vi "Execute Industrial Controllers.vi"(8 "error in (no error)":errorcluster, 11 "State Variables in":T1 {"Config"."Config"."Industrial Settings"."Write Refs"."Data Reference" format="%.0x"; "Config"."Config"."Industrial Settings"."Read Refs"."Data Reference" format="%.0x"; "Config"."Config"."PID Settings"."Read Refs"."Data Reference" format="%.0x"; "Config"."Config"."PID Settings"."Write Refs"."Data Reference" format="%.0x"}) -> (0 "error out":errorcluster, 3 "State Variables out":T1 {"Config"."Config"."Industrial Settings"."Write Refs"."Data Reference" format="%.0x"; "Config"."Config"."Industrial Settings"."Read Refs"."Data Reference" format="%.0x"; "Config"."Config"."PID Settings"."Read Refs"."Data Reference" format="%.0x"; "Config"."Config"."PID Settings"."Write Refs"."Data Reference" format="%.0x"})   [LabVIEW 2015, in "Control Addon Engine.lvlib"]
uses:
  Control Addon Engine.lvlib
  Types/RT Driver State Variables.ctl
  <vilib>/NI/NIVS Inline Async API/_VS Inline Async API/VS Inline Async API/VS Inline Async API.lvclass
  Types/RT Configuration.ctl
  Shared/Types/Gain Schedule.ctl
  Shared/Types/Compiled Settings.ctl
  Shared/Types/Compiled PID Settings.ctl
  <vilib>/NI Veristand/Custom Device API/Block Data Reference.ctl
  <vilib>/NI Veristand/Custom Device API/Data Reference.ctl
  Shared/Types/Compiled Industrial Settings.ctl
  Shared/Types/Compiled Industrial Parameters.ctl
  <vilib>/NI Veristand/Custom Device API/Global Data Refs.vi
  <vilib>/NI VeriStand/Custom Device API/Custom Device API.lvlib
  Shared/Control Addon Shared.lvlib
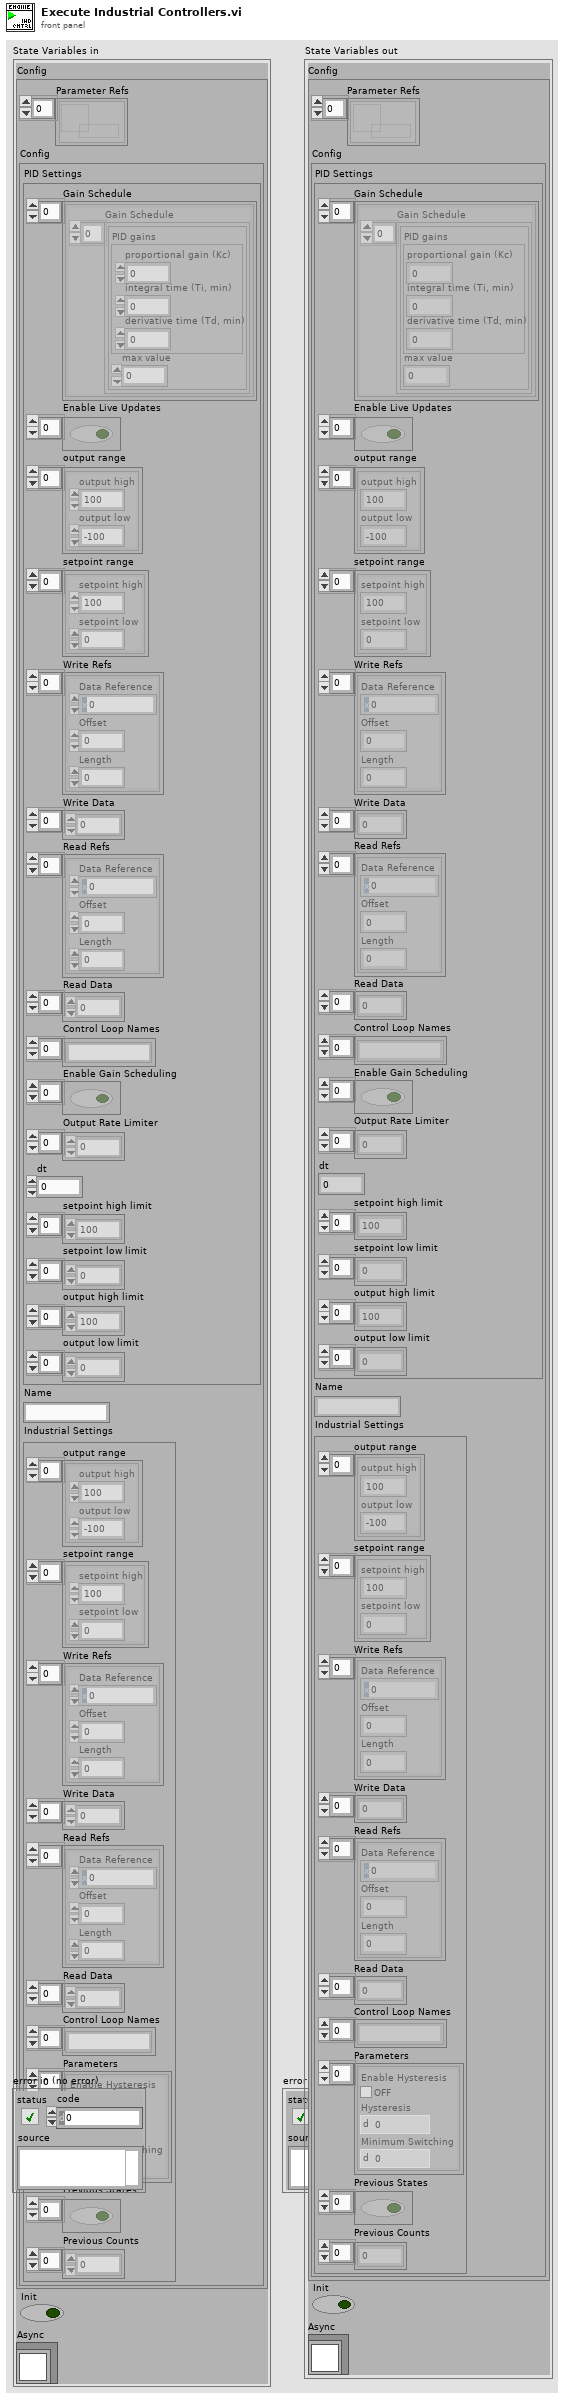
[diagram p1: front panel]
types:
  T1 = typedef "Control Addon Engine.lvlib/RT Driver State Variables.ctl" = cluster{"Config":T2, "Init":bool, "Async":refnum<class "VS Inline Async API.lvclass">}
  T2 = typedef "Control Addon Engine.lvlib/RT Configuration.ctl" = cluster{"Parameter Refs":refnum<data-value>[], "Config":T3}
  T3 = typedef "Control Addon Shared.lvlib/Compiled Settings.ctl" = cluster{"PID Settings":T4, "Name":string, "Industrial Settings":T8}
  T4 = typedef "Control Addon Shared.lvlib/Compiled PID Settings.ctl" = cluster{"Gain Schedule":T5[], "Enable Live Updates":bool[], "output range":cluster{"output high":dbl, "output low":dbl}[], "setpoint range":cluster{"setpoint high":dbl, "setpoint low":dbl}[], "Write Refs":T6[], "Write Data":dbl[], "Read Refs":T6[], "Read Data":dbl[], "Control Loop Names":string[], "Enable Gain Scheduling":bool[], "Output Rate Limiter":dbl[], "dt":dbl, "setpoint high limit":dbl[], "setpoint low limit":dbl[], "output high limit":dbl[], "output low limit":dbl[]}
  T5 = typedef "Control Addon Shared.lvlib/Gain Schedule.ctl" = cluster{"Gain Schedule":cluster{"PID gains":cluster{"proportional gain (Kc)":dbl, "integral time (Ti, min)":dbl, "derivative time (Td, min)":dbl}, "max value":dbl}[]}
  T6 = typedef "Custom Device API.lvlib/Block Data Reference.ctl" = cluster{"Data Reference":T7, "Offset":u64, "Length":u64}
  T7 = typedef "Custom Device API.lvlib/Data Reference.ctl" = i32
  T8 = typedef "Control Addon Shared.lvlib/Compiled Industrial Settings.ctl" = cluster{"output range":cluster{"output high":dbl, "output low":dbl}[], "setpoint range":cluster{"setpoint high":dbl, "setpoint low":dbl}[], "Write Refs":T6[], "Write Data":dbl[], "Read Refs":T6[], "Read Data":dbl[], "Control Loop Names":string[], "Parameters":T9[], "Previous States":bool[], "Previous Counts":u64[]}
  T9 = typedef "Control Addon Shared.lvlib/Compiled Industrial Parameters.ctl" = cluster{"Enable Hysteresis":bool, "Hysteresis":dbl, "Minimum Switching":u64}
  T10 = cluster{"setpoint high":dbl, "setpoint low":dbl}[]
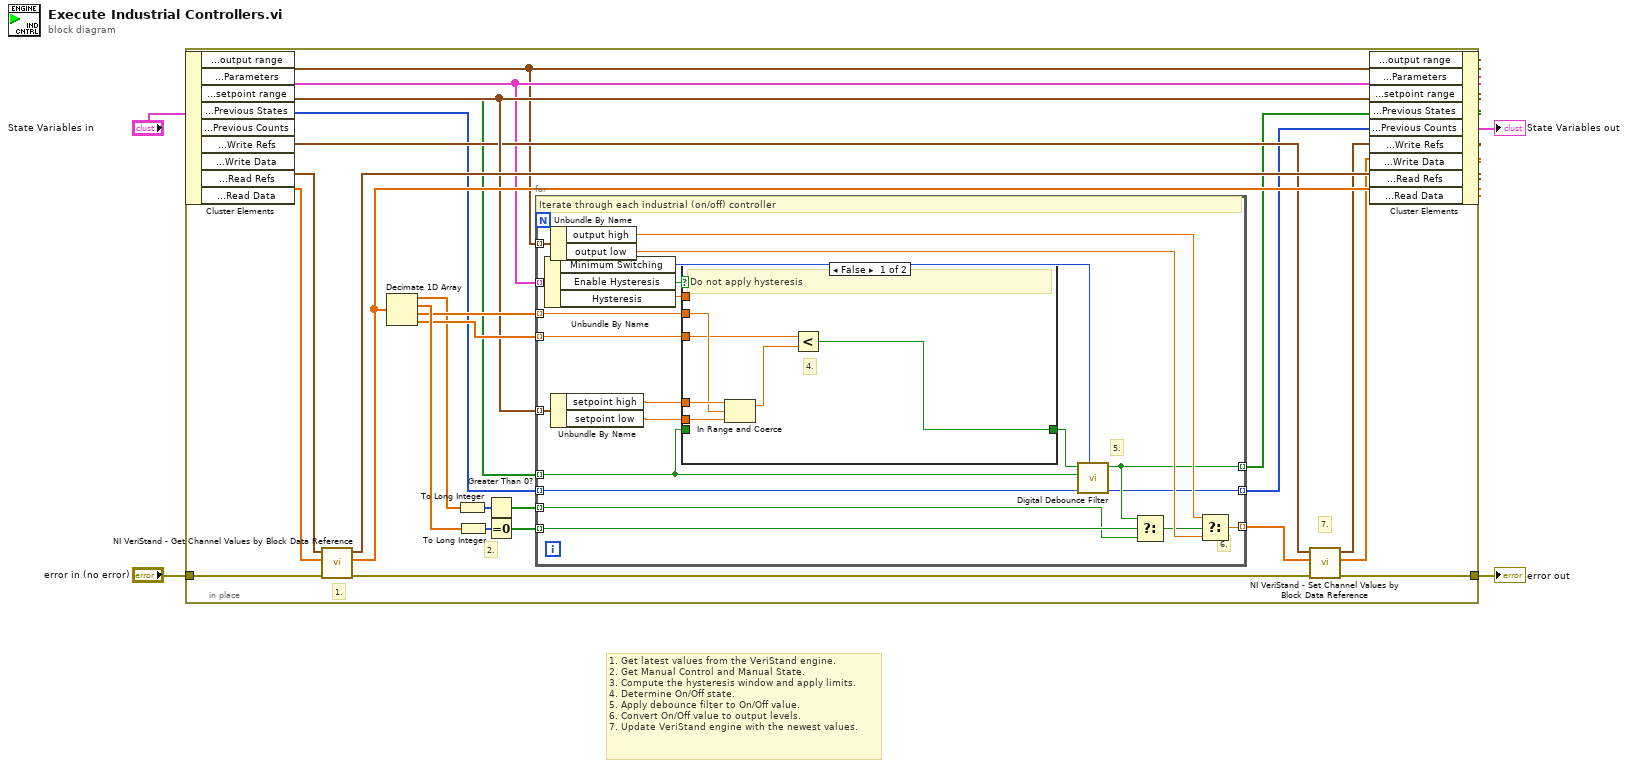
[diagram p0: block diagram]
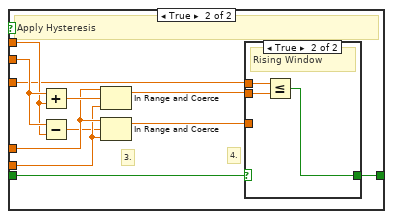
[diagram p2: hidden frame]
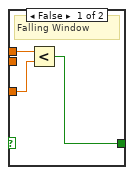
[diagram p3: hidden frame]
diagram:
  # "1. Get latest values from the VeriStand engine.\n2. Get Manual Control and Manual State.\n3. Compute the hysteresis window and apply limits.\n4. Determine On/Off state.\n5. Apply debounce filter to On/Off value.\n6. Convert On/Off value to output levels.\n7. Update VeriStand engine with the newest values."
  n1 = in-place {
    in-place-border: "error in (no error)" -> [w30]
    in-place-border: [w18] -> w4
    # "7."
    # "2."
    # "1."
    n2 = in-place-cluster #1("State Variables in") -> ("Config.Config.Industrial Settings.output range"=w5:cluster{"output high":dbl, "output low":dbl}[], "Config.Config.Industrial Settings.Parameters"=w10:T9[], "Config.Config.Industrial Settings.setpoint range"=w19:T10, "Config.Config.Industrial Settings.Previous States"=w9:bool[], "Config.Config.Industrial Settings.Previous Counts"=w8:u64[], "Config.Config.Industrial Settings.Write Refs"=w17:T6[], "Config.Config.Industrial Settings.Read Refs"=w29:T6[], "Config.Config.Industrial Settings.Read Data"=w28:dbl[])  [unwired: 1 out]
    n3 = call <vilib>:"NI VeriStand - Get Channel Values by Block Data Reference.vi"("error in (no error)"=w30, "Values Array in"=w28, "Block Data Ref"=w29) -> ("error out"=w25:errorcluster, "Values Array out"=w24:dbl[], "Block Data Ref dup"=w26:T6[])  [unwired: 6 in]
    n4 = Decimate 1D Array(w24) -> (w12:dbl[], w22:dbl[], w21:dbl[], w20:dbl[])
    n5 = To Long Integer(number=w12) -> (32bit integer=w13:i32[])
    n6 = To Long Integer(number=w22) -> (32bit integer=w27:i32[])
    n7 = Greater Than 0?(x=w13) -> (x > 0?=w11:bool[])
    n8 = Equal To 0?(x=w27) -> (x = 0?=w23:bool[])
    n9 = for {
      tunnel: w11 -> [w48] mode=indexing
      tunnel: w23 -> [w51] mode=indexing
      tunnel: w21 -> [w42] mode=indexing
      tunnel: w20 -> [w38] mode=indexing
      tunnel: w19 -> [w50] mode=indexing
      tunnel: w5 -> [w49] mode=indexing
      tunnel: [w44] -> w14 mode=indexing
      tunnel: w10 -> [w43] mode=indexing
      tunnel: w9 -> [w34] mode=indexing
      tunnel: [w36] -> w7 mode=indexing
      tunnel: w8 -> [w33] mode=indexing
      tunnel: [w32] -> w6 mode=indexing
      # "6."
      # "5."
      # "Iterate through each industrial (on/off) controller"
      n10 = Unbundle By Name(w43) -> ("Minimum Switching"=w31:u64, "Enable Hysteresis"=w37:bool, "Hysteresis"=w41:dbl)
      n11 = Unbundle By Name(w49) -> ("output high"=w46:dbl, "output low"=w47:dbl)
      n12 = Unbundle By Name(w50) -> ("setpoint high"=w40:dbl, "setpoint low"=w39:dbl)
      n13 = case shown="False" w37 {
        tunnel: w42 -> [w55 w68]
        tunnel: w41 -> [_ w67]
        tunnel: w40 -> [w57 w65]
        tunnel: w39 -> [w56 w64]
        tunnel: w38 -> [w53 w62]
        tunnel: [w52 w61] -> w35
        tunnel: w34 -> [_ w58]
        frame False {
          # "4."
          # "Do not apply hysteresis"
          n14 = In Range and Coerce(upper limit=w57, x=w55, lower limit=w56) -> (coerced(x)=w54:dbl)  [unwired: 1 out]
          n15 = Less?(x=w53, y=w54) -> (x < y?=w52:bool)
        }
        frame True {
          # "4."
          # "3."
          # "Apply Hysteresis"
          n16 = Add(x=w68, y=w67) -> (x+y=w66:dbl)
          n17 = Subtract(x=w68, y=w67) -> (x-y=w63:dbl)
          n18 = In Range and Coerce(upper limit=w65, x=w66, lower limit=w64) -> (coerced(x)=w60:dbl)  [unwired: 1 out]
          n19 = In Range and Coerce(upper limit=w65, x=w63, lower limit=w64) -> (coerced(x)=w59:dbl)  [unwired: 1 out]
          n20 = case shown="True" w58 {
            tunnel: w62 -> [w71 w74]
            tunnel: [w69 w73] -> w61
            tunnel: w60 -> [_ w72]
            tunnel: w59 -> [w70 _]
            frame False {
              # "Falling Window"
              n21 = Less?(x=w71, y=w70) -> (x < y?=w69:bool)
            }
            frame True {
              # "Rising Window"
              n22 = Less Or Equal?(x=w74, y=w72) -> (x <= y?=w73:bool)
            }
          }
        }
      }
      n23 = call "Digital Debounce Filter.vi"("Cycles to Filter"=w31, "Previous Count"=w33, "Previous Input Signal"=w34, "Input Signal"=w35) -> ("Count"=w32:u64, "Output Filtered Signal"=w36:bool)  [unwired: 6 in]
      n24 = Select(t=w36, s=w51, f=w48) -> (s? t:f=w45:bool)
      n25 = Select(t=w46, s=w45, f=w47) -> (s? t:f=w44:dbl)
    }
    n26 = call <vilib>:"NI VeriStand - Set Channel Values by Block Data Reference.vi"("error in (no error)"=w25, "Values Array in"=w14, "Block Data Ref"=w17) -> ("error out"=w18:errorcluster, "Values Array out"=w16:dbl[], "Block Data Ref dup"=w15:T6[])  [unwired: 6 in]
    n27 = in-place-cluster #1("Config.Config.Industrial Settings.output range"=w5, "Config.Config.Industrial Settings.Parameters"=w10, "Config.Config.Industrial Settings.setpoint range"=w19, "Config.Config.Industrial Settings.Previous States"=w7, "Config.Config.Industrial Settings.Previous Counts"=w6, "Config.Config.Industrial Settings.Write Refs"=w15, "Config.Config.Industrial Settings.Write Data"=w16, "Config.Config.Industrial Settings.Read Refs"=w26, "Config.Config.Industrial Settings.Read Data"=w24) -> (→"State Variables out":T1)
  }
  "error out" <- w4
